vi "Subvi_Online_SVM_SWLDA_newMethod_in_분석기.vi"(0 "rate":dbl=500.0 caption="Rate" format="%0.2f", 1 "samples per channel":i32=25, 2 "in":T1, 4 "Brain_data_source":dbl[][](array[numeric]) caption="EEG_Raw_Data" format="%0.3f", 5 "Target_Flash_Order":i64[][](array[numeric]), 6 "Value":T1, 7 "svm_model_file":string, 8 "Matrix":T1, 10 "Target":path, 12 "Nontarget":path) -> (13 "EPR_발생_total":i16[](array[numeric]), 14 "output-0~8":i32, 15 "decision":dbl[](array[numeric]), 18 "SWLDA":dbl[](array[numeric]), 19 "ERP_Parameters":dbl[][](array[numeric]))   [LabVIEW 2014]
uses:
  <vilib>/Analysis/Matrix/Datatypes/RealMatrix.ctl
  <vilib>/Analysis/3filter.llb/Filter Passband Type.ctl
  <vilib>/Analysis/baseanly.llb/Mean (DBL).vi
  <vilib>/Analysis/3filter.llb/Butterworth Filter (DBL).vi
  <vilib>/Utility/file.llb/Read From Spreadsheet File (DBL).vi
  <vilib>/Analysis/Matrix/Numeric/Conversions/Array To Matrix - RA.vi
  <vilib>/Analysis/Matrix/Numeric/Multiply/Multiply - RM,RM.vi
  <vilib>/Analysis/Matrix/Numeric/Subtract/Subtract - RM,RM.vi
  <vilib>/Analysis/Matrix/Numeric/Conversions/Matrix To Array - RM.vi
  <vilib>/Analysis/NI_AALBase.lvlib
  <vilib>/Analysis/Matrix/NI_Matrix.lvlib
  <vilib>/Analysis/Matrix/Numeric/Conversions/Array To Matrix - RA2.vi
panel:
  out "Real":dbl
  out "deleted portion":dbl[][](array[numeric])
  out "2-D Array of Real 3":dbl[][](array[numeric])
  out "2-D Array of Real 2":dbl[][](array[numeric])
  out "2-D Array of Real":dbl[][](array[numeric])
  out "1-D Array of Real":dbl[](array[numeric])
  out "SWLDA_original":dbl[][](array[numeric])
  out "size(s)":i32[](array[numeric])
  in  "LDA":path=path "C:/Users/Administrator/Desktop/공공복지안전사업연구-노수진/파일럿20130902/LDA_Matrix_Value.xls"
  out "전치된 배열":dbl[][](array[numeric])
  out "#channel":i32
  out "#sti 6":i32
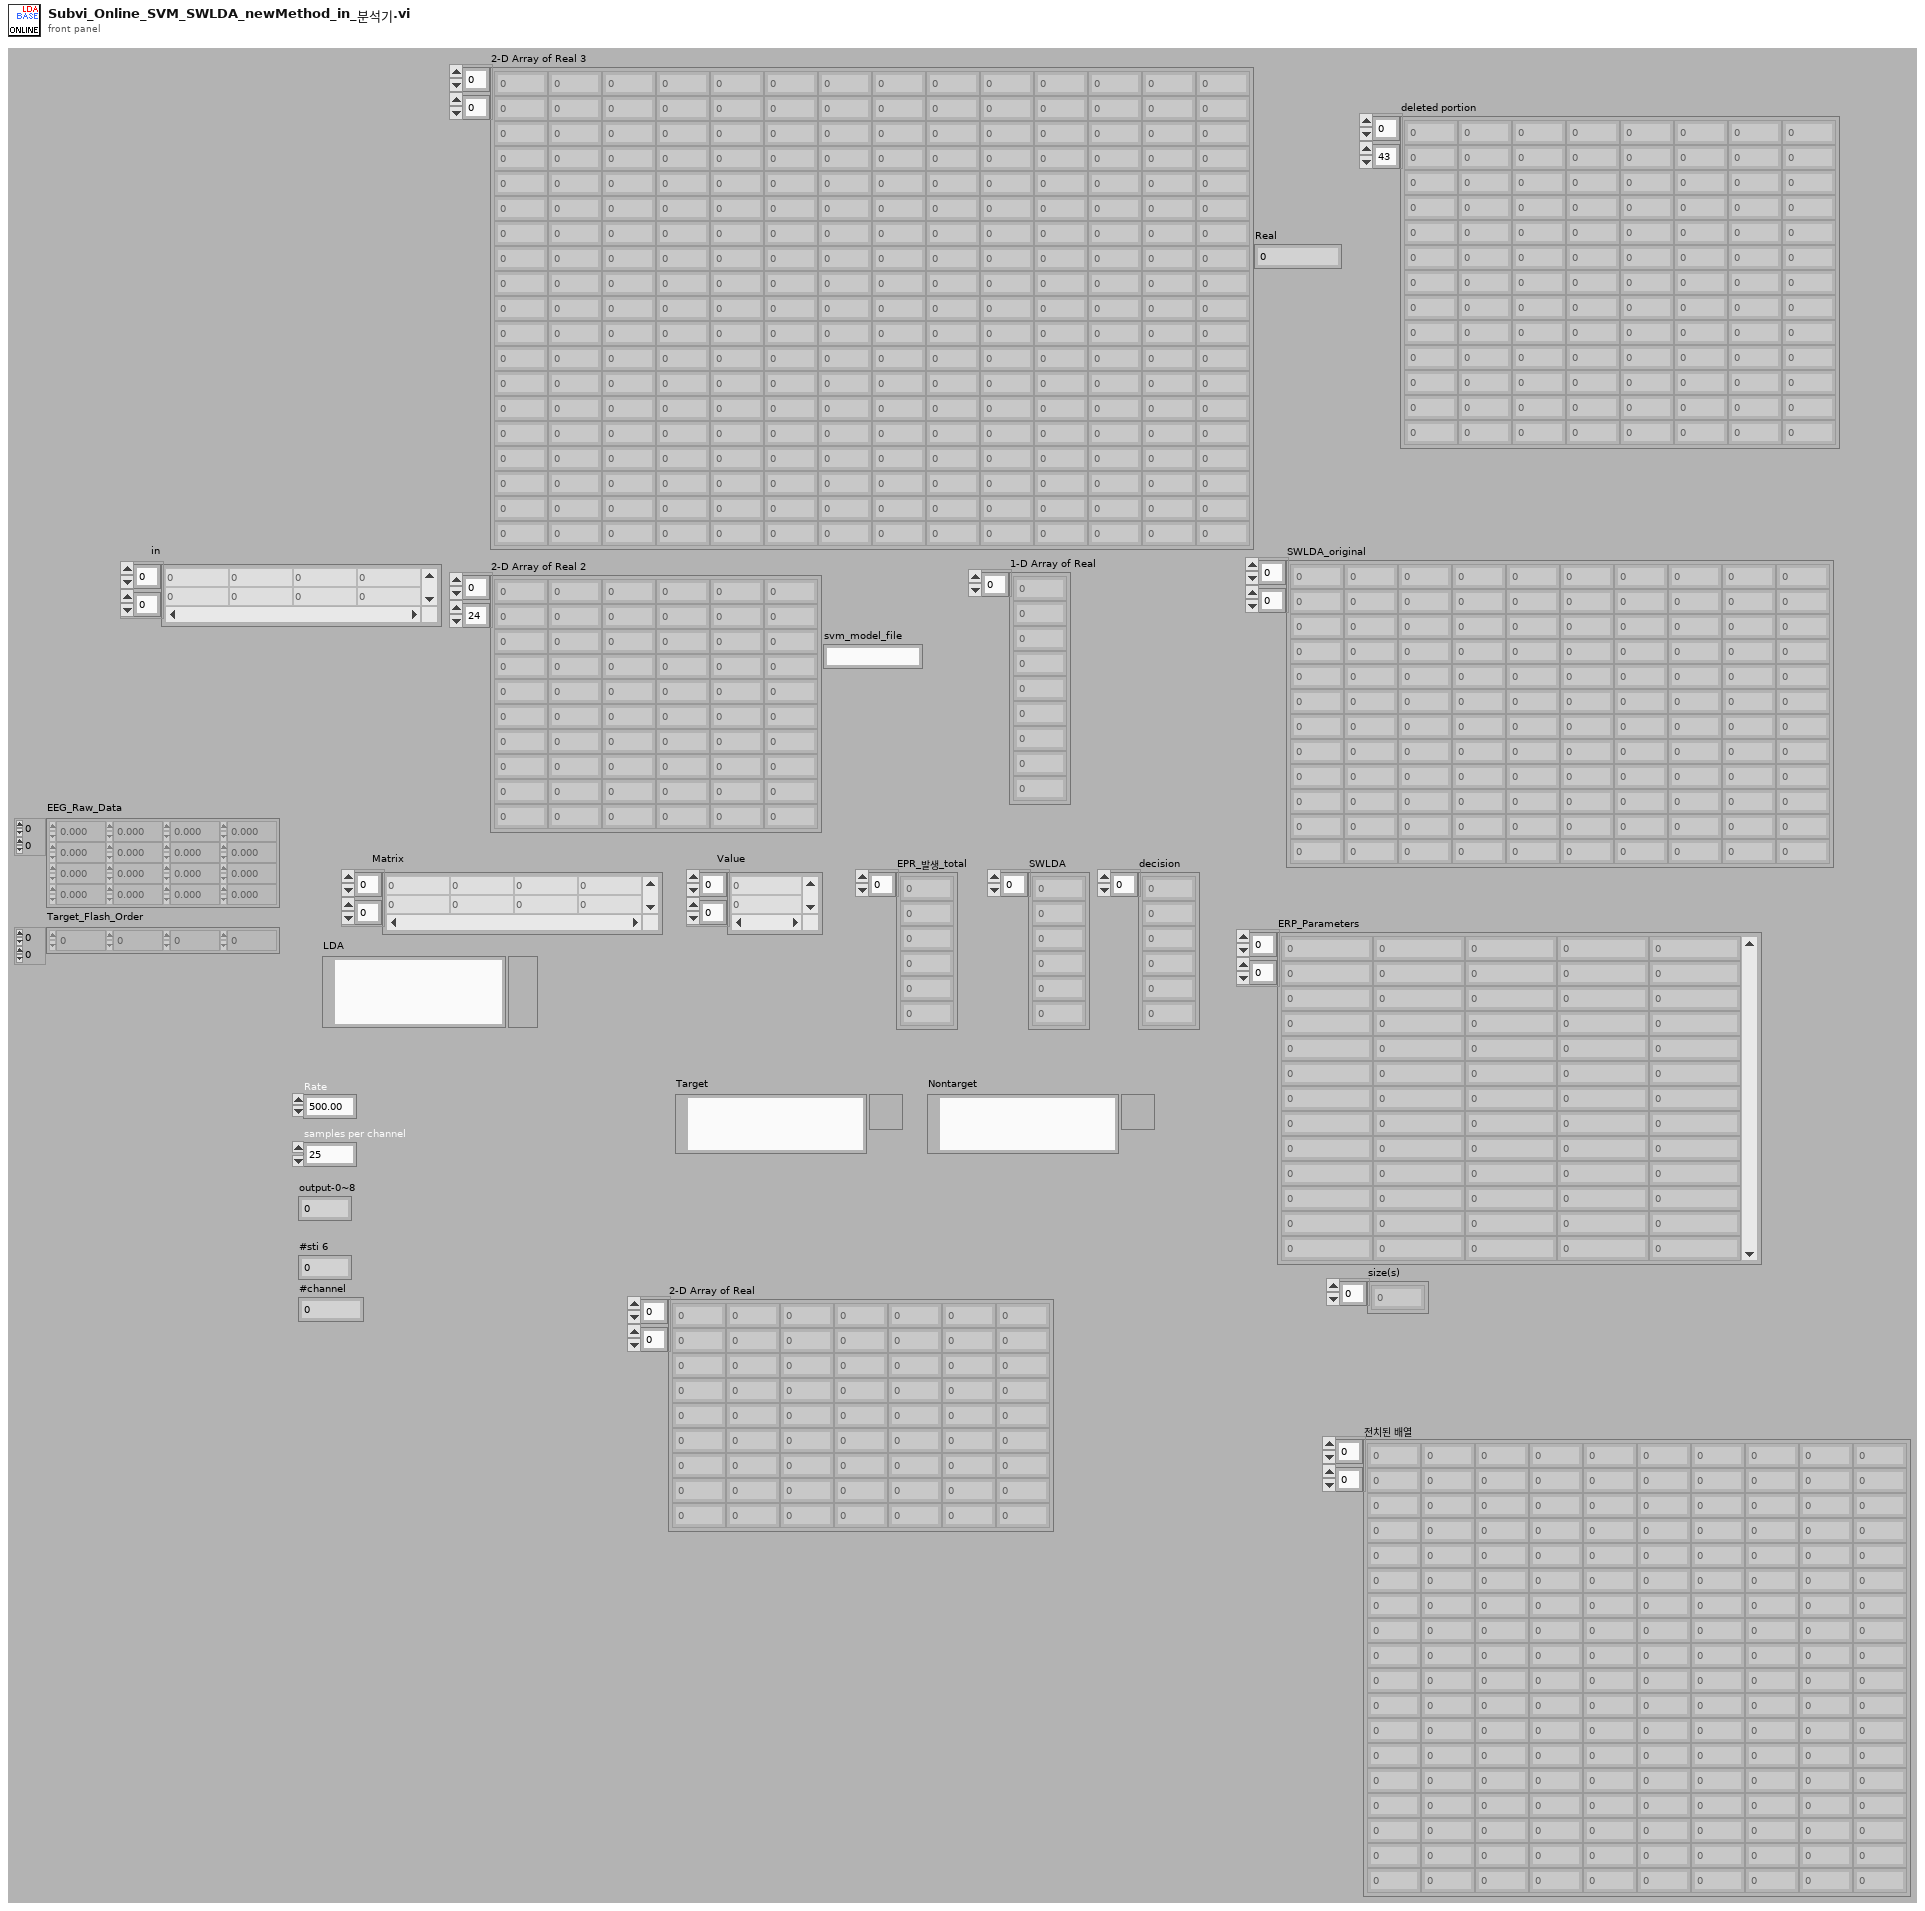
[diagram p1: front panel]
types:
  T1 = typedef "NI_Matrix.lvlib/RealMatrix.ctl" = dbl[][]
  T2 = typedef "NI_AALBase.lvlib/Filter Passband Type.ctl" = enum32{"Lowpass", "Highpass", "Bandpass", "Bandstop"}
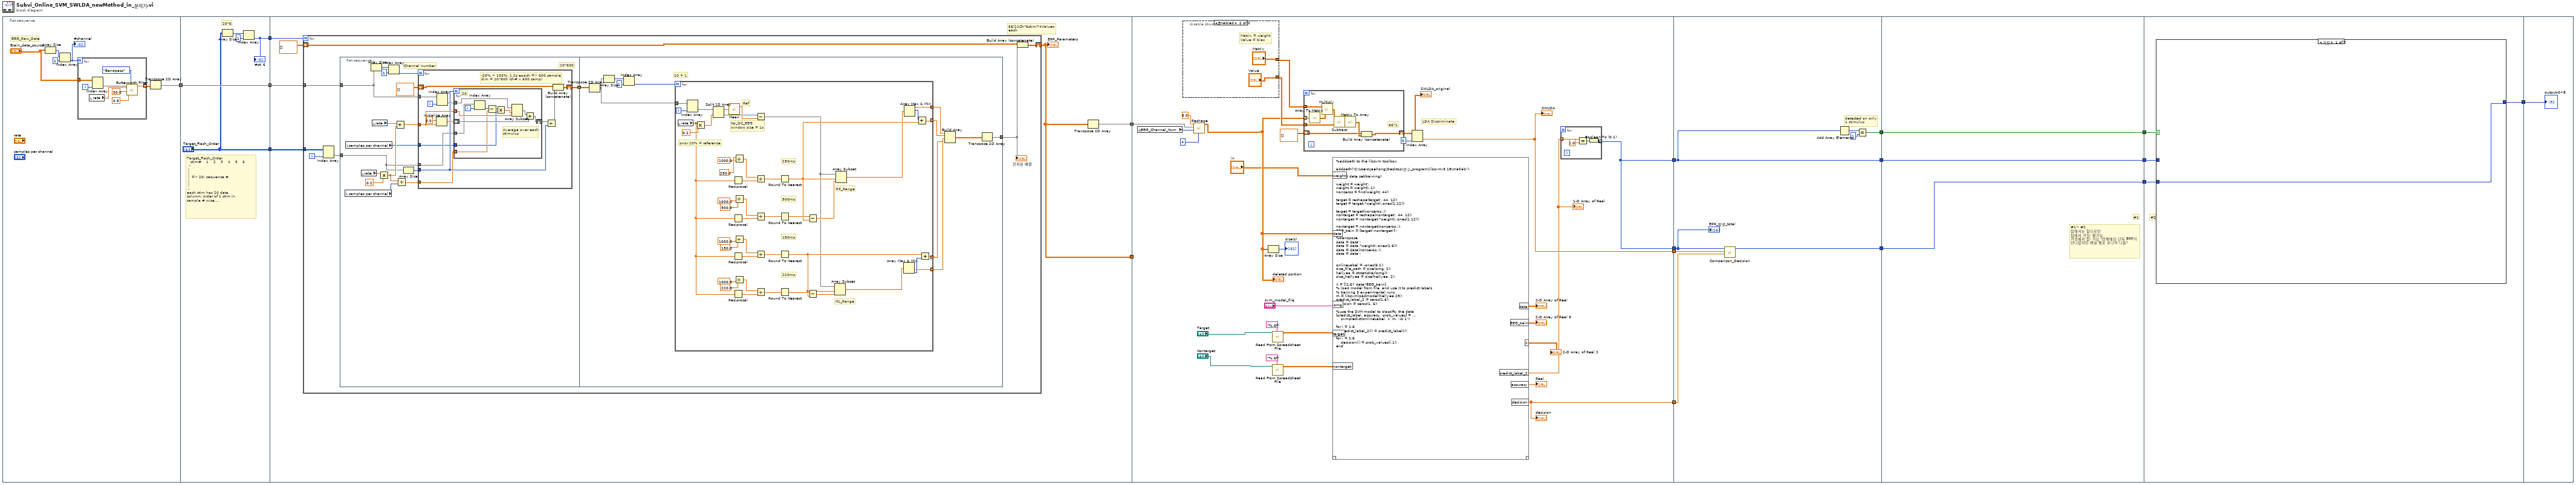
[diagram p0: block diagram]
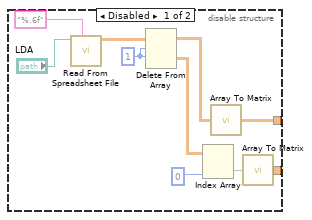
[diagram p2: hidden frame]
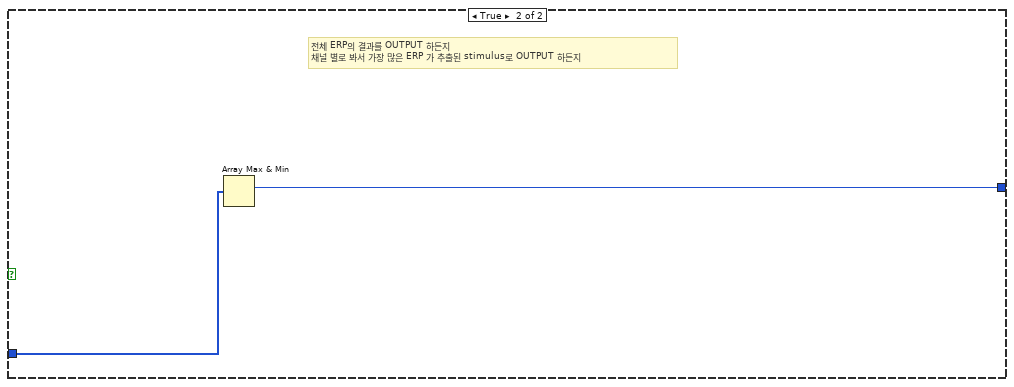
[diagram p3: hidden frame]
diagram:
  n1 = flat-sequence {
    tunnel: [w19] -> w17
    tunnel: [w36] -> w16
    tunnel: ["Target_Flash_Order"] -> w15
    tunnel: w17 -> [w36]
    tunnel: [w33] -> w14
    tunnel: w16 -> [w42]
    tunnel: w15 -> [w41]
    tunnel: w14 -> [w40]
    tunnel: [w37] -> w13
    tunnel: [w38] -> w12
    tunnel: w13 -> [w157]
    tunnel: w12 -> [_]
    tunnel: [w171] -> w11
    tunnel: [w171] -> w9
    tunnel: [w168] -> w7
    tunnel: [w152] -> w3
    tunnel: w11 -> [w204]
    tunnel: [w205] -> w10
    tunnel: w9 -> [w203]
    tunnel: w7 -> [w202]
    tunnel: [w204] -> w6
    tunnel: w3 -> [w201]
    tunnel: [w200] -> w2
    tunnel: w10 -> [w209]
    tunnel: w6 -> [w210]
    tunnel: [w210] -> w5
    tunnel: [w209] -> w4
    tunnel: w2 -> [w208]
    tunnel: [w208] -> w1
    tunnel: [w214] -> w8
    tunnel: w5 -> [w212]
    tunnel: w4 -> [w213]
    tunnel: w1 -> [w211]
    tunnel: w8 -> [w218]
    frame #0 {
      # "EEG_Raw_Data"
      n2 = Array Size(array="Brain_data_source") -> (size(s)=w20:i32[])
      n3 = Index Array(array=w20, index=1) -> (element=w22:i32)
      "#channel" <- w22
      n4 = for {
        N: w22 -> [_]
        tunnel: "Brain_data_source" -> [w31]
        tunnel: [w27] -> w23 mode=indexing
        i -> [w30]
        n5 = local read "rate"() -> (w24:dbl)
        n6 = Index Array(array=w31, index (col)=w30) -> (element=w29:dbl[])  [unwired: 1 in]
        n7 = call-poly <vilib>:"Butterworth Filter.vi"("filter type"=Filter_Passband_Type."Bandpass", "low cutoff freq: fl"=0.5, "high cutoff freq: fh"=30.0, "sampling freq: fs"=w24, "X"=w29) -> ("Filtered X"=w27:dbl[])  [unwired: 3 in, 1 out]
      }
      n8 = Transpose 2D Array(2D array=w23) -> (transposed array=w19:dbl[][])
    }
    frame #1 {
      # "Target_Flash_Order\n   stim#    1    2    3    4    5    6    \n  -\n |\n |\n |  => 20: sequence # \n |\n |\n -\neach stim has 20 data\ncolumn: order of 1 stim in \nsample # wise...."
      # "20*6"
      n9 = Array Size(array="Target_Flash_Order") -> (size(s)=w35:i32[])
      n10 = Index Array(array=w35, index=1 ("인덱스")) -> (element=w33:i32)
      "#sti 6" <- w33
    }
    frame #2 {
      # "66(11Ch*6stim)*4Values\neach"
      n11 = for {
        N: w40 -> [_]
        tunnel: w42 -> [w49]
        tunnel: w41 -> [w48]
        shift-right: [w45] -> w38
        shift-left: dbl[][] [] -> [w44]
        i -> [w47]
        n12 = Index Array(array=w48, index (col)=w47) -> (element=w46:i64[])  [unwired: 1 in]
        n13 = flat-sequence {
          tunnel: w49 -> [w53]
          tunnel: w46 -> [w52]
          tunnel: [w51] -> w50
          tunnel: w50 -> [w97]
          tunnel: [w93] -> w43
          frame #0 {
            # "10*600"
            # "Channel number"
            n14 = local read "samples per channel"() -> (w60:i32)
            n15 = local read "samples per channel"() -> (w59:i32)
            n16 = local read "rate"() -> (w62:dbl)
            n17 = Array Size(array=w53) -> (size(s)=w56:i32[])
            n18 = local read "rate"() -> (w64:dbl)
            n19 = Multiply(x=w62, y=0.2) -> (x*y=w66:dbl)
            n20 = Index Array(array=w56, index=1) -> (element=w58:i32)
            n21 = Add(x=w64, y=w66) -> (x+y=w65:dbl)
            n22 = Divide(x=w66, y=w60) -> (x/y=w63:dbl)
            n23 = Array Size(array=w52) -> (size(s)=w55:i32)
            n24 = for {
              N: w58 -> [_]
              tunnel: w59 -> [w67]
              tunnel: w65 -> [w78]
              shift-right: [w71] -> w51
              shift-left: dbl[][] [] -> [w73]
              tunnel: w55 -> [w72]
              tunnel: w53 -> [w70]
              tunnel: w52 -> [w69]
              tunnel: w63 -> [w68]
              i -> [w80]
              # "-20% ~ 100%: 1.2s epoch => 600 sample\ndim = 10*600 (ch# x 600 samp)"
              n25 = Initialize Array(0.0 ("element"), w78) -> (w77:dbl[])
              n26 = Index Array(array=w70, index (col)=w80) -> (element=w79:dbl[])  [unwired: 1 in]
              n27 = for {
                N: w72 -> [_]
                tunnel: w79 -> [w92]
                shift-right: [w89] -> w75
                shift-left: w77 -> [w90]
                tunnel: w78 -> [w88]
                tunnel: w69 -> [w86]
                tunnel: w68 -> [w84]
                tunnel: w67 -> [w82]
                i -> [w87]
                # "Average over each\nstimulus"
                # "20"
                n28 = Index Array(array=w86, index=w87) -> (element=w85:i64)
                n29 = Subtract(x=w85, y=w84) -> (x-y=w83:dbl)
                n30 = Multiply(x=w83, y=w82) -> (x*y=w81:dbl)
                n31 = Array Subset(array=w92, index=w81, length=w88) -> (w91:dbl[])
                n32 = Add(x=w91, y=w90) -> (x+y=w89:dbl[])
              }
              n33 = Divide(x=w75, y=w72) -> (x/y=w74:dbl[])
              n34 = Build Array (concatenate)(w73, w74) -> (w71:dbl[][])
            }
          }
          frame #1 {
            # "10 + 1"
            n35 = Transpose 2D Array(2D array=w97) -> (transposed array=w95:dbl[][])
            n36 = Array Size(array=w95) -> (size(s)=w98:i32[])
            n37 = Index Array(array=w98, index=1) -> (element=w94:i32)
            n38 = for {
              N: w94 -> [_]
              tunnel: w95 -> [w147]
              tunnel: [w142] -> w102 mode=indexing
              tunnel: [w140] -> w101 mode=indexing
              tunnel: [w111] -> w100 mode=indexing
              tunnel: [w137] -> w99 mode=indexing
              i -> [w136]
              # "P3_Range"
              # "N1_Range"
              # "220ms"
              # "150ms"
              # "500ms"
              # "250ms"
              # "No_DC_EEG\nwindow size = 1s"
              # "Ref"
              # "prior 20% = reference"
              n39 = local read "rate"() -> (w118:dbl)
              n40 = Index Array(array=w147, index (col)=w136) -> (element=w139:dbl[])  [unwired: 1 in]
              n41 = Multiply(x=w118, y=0.2) -> (x*y=w145:dbl)
              n42 = Split 1D Array(array=w139, index=w145) -> (first subarray=w144:dbl[], second subarray=w135:dbl[])
              n43 = call-poly <vilib>:"Mean.vi"("X"=w144) -> ("mean"=w143:dbl)  [unwired: 1 out]
              n44 = Reciprocal(x=w118) -> (1/x=w134:dbl)
              n45 = Reciprocal(x=w118) -> (1/x=w133:dbl)
              n46 = Reciprocal(x=w118) -> (1/x=w132:dbl)
              n47 = Reciprocal(x=w118) -> (1/x=w131:dbl)
              n48 = Divide(x=250.0, y=1000.0) -> (x/y=w130:dbl)
              n49 = Divide(x=500.0, y=1000.0) -> (x/y=w129:dbl)
              n50 = Divide(x=150.0, y=1000.0) -> (x/y=w128:dbl)
              n51 = Divide(x=220.0, y=1000.0) -> (x/y=w127:dbl)
              n52 = Subtract(x=w135, y=w143) -> (x-y=w104:dbl[])
              n53 = Divide(x=w130, y=w134) -> (x/y=w117:dbl)
              n54 = Divide(x=w129, y=w133) -> (x/y=w116:dbl)
              n55 = Divide(x=w128, y=w132) -> (x/y=w115:dbl)
              n56 = Divide(x=w127, y=w131) -> (x/y=w114:dbl)
              n57 = Round To Nearest(number=w117) -> (nearest integer value=w107:dbl)
              n58 = Round To Nearest(number=w116) -> (nearest integer value=w113:dbl)
              n59 = Round To Nearest(number=w115) -> (nearest integer value=w109:dbl)
              n60 = Round To Nearest(number=w114) -> (nearest integer value=w112:dbl)
              n61 = Subtract(x=w113, y=w107) -> (x-y=w108:dbl)
              n62 = Subtract(x=w112, y=w109) -> (x-y=w110:dbl)
              n63 = Array Subset(array=w104, index=w109, length=w110) -> (w105:dbl[])
              n64 = Array Subset(array=w104, index=w107, length=w108) -> (w106:dbl[])
              n65 = Array Max & Min(array=w105) -> (min value=w111:dbl, min index (indices)=w138:i32)  [unwired: 2 out]
              n66 = Array Max & Min(array=w106) -> (max value=w142:dbl, max index (indices)=w141:i32)  [unwired: 2 out]
              n67 = Add(x=w141, y=w107) -> (x+y=w140:dbl)
              n68 = Add(x=w109, y=w138) -> (x+y=w137:dbl)
            }
            n69 = Build Array(w102, w101, w100, w99) -> (w96:dbl[][])
            n70 = Transpose 2D Array(2D array=w96) -> (transposed array=w93:dbl[][])
          }
        }
        n71 = Build Array (concatenate)(w44, w43) -> (w45:dbl[][])
        "전치된 배열" <- w43
      }
      "ERP_Parameters" <- w38
      n72 = Transpose 2D Array(2D array=w38) -> (transposed array=w37:dbl[][])
    }
    frame #3 {
      # "LDA Discriminate"
      # "66*1"
      n73 = global read "Control_Panel_정리.vi" "EEG_Channel_Num"() -> (w156:i32)
      n74 = disable-structure shown="Enabled" {
        disable-tunnel: [w179 "Matrix"] -> w169
        disable-tunnel: [w178 "Value"] -> w170
        frame Disabled {
          w181 = 1 ("인덱스 (행)")
          n75 = call-poly <vilib>:"Read From Spreadsheet File.vi"("format (%.3f)"="%.6f", "file path (dialog if empty)"="LDA") -> ("all rows"=w175:dbl[][])  [unwired: 5 in, 4 out]
          n76 = Delete From Array(array=w175, length=w181, index (row)=w181) -> (deleted portion=w184:dbl[][], array with subset deleted=w183:dbl[][])  [unwired: 1 in]
          n77 = Index Array(array=w184, index (col)=0 ("인덱스")) -> (element=w182:dbl[])  [unwired: 1 in]
          n78 = call-poly <vilib>:"Array To Matrix.vi"("Real 2D Array"=w183) -> ("Real Matrix"=w179:T1)
          n79 = call-poly <vilib>:"Array To Matrix.vi"("Real 1D Array"=w182) -> ("Real Matrix (Column Vector)"=w178:T1)
        }
        frame Enabled {
          # "Matrix = weight\nValue = bias"
        }
      }
      n80 = call "Reshape.vi"("Numeric"=4, "EEG_Channel_Num"=w156, "all rows"=w157, "Numeric 2"=6.0) -> ("Array"=w153:dbl[][])  [unwired: 7 in]
      "deleted portion" <- w153
      n81 = Array Size(array=w153) -> (size(s)=→"size(s)":i32[])
      n82 = call-poly <vilib>:"Read From Spreadsheet File.vi"("format (%.3f)"="%.6f", "file path (dialog if empty)"="Target") -> ("all rows"=w165:dbl[][])  [unwired: 5 in, 4 out]
      n83 = call-poly <vilib>:"Read From Spreadsheet File.vi"("format (%.3f)"="%.6f", "file path (dialog if empty)"="Nontarget") -> ("all rows"=w164:dbl[][])  [unwired: 5 in, 4 out]
      n84 = for {
        tunnel: w169 -> [w191]
        tunnel: w170 -> [w197]
        shift-right: [w194] -> w172
        shift-left: dbl[][] [] -> [w193]
        tunnel: w153 -> [w192] mode=indexing
        n85 = call-poly <vilib>:"Array To Matrix.vi"("Real 1D Array"=w192) -> ("Real Matrix (Column Vector)"=w196:T1)
        n86 = call-poly <vilib>:"Multiply.vi"("Real Matrix B"=w196, "Real Matrix A"=w191) -> ("A * B"=w199:T1)
        n87 = call-poly <vilib>:"Subtract.vi"("Real Matrix B"=w197, "Real Matrix A"=w199) -> ("A - B"=w198:T1)
        n88 = call-poly <vilib>:"Matrix To Array.vi"("Real Matrix"=w198) -> ("Real 2D Array"=w195:dbl[][])
        n89 = Build Array (concatenate)(w193, w195) -> (w194:dbl[][])
      }
      "SWLDA_original" <- w172
      n90 = script code="%addpath to the libsvm toolbox\n\naddpath('C:\\Users\\Jaehong\\Desktop\\연구_program\\libsvm-3.18\\matlab');\n\n%read data set(training)\n\nweight = weight';\nweight = weight(:,1);\nnonzeros = find(weight, 44);\n\ntarget = reshape(target', 44, 12);\ntarget = target.*weight(:,ones(1,12));\n\ntarget = target(nonzeros,:);\nnontarget = reshape(nontarget', 44, 12);\nnontarget = nontarget.*weight(:,ones(1,12));\n\nnontarget = nontarget(nonzeros,:);\nEEG_train = [target';nontarget']';\n\n%transpose\ndata = data';\ndata = data.*weight(:,ones(1,6));\ndata = data(nonzeros,:);\ndata = data';\n\n\nonlineLabel = -ones(6,1);\nsize_file_path = size(omg, 2);\nhellyea = strcat(char(omg));\nsize_hellyea = size(hellyea, 2);\n\nX = [(1:6)' data*EEG_train];\n% load model from file, and use it to predict labels\n% training 3 experimental runs\nm = libsvmloadmodel(hellyea,25);\npredict_label_2 = zeros(1,6);\ndecision = zeros(1, 6);\n\n%use the SVM model to classifty the data\n[predict_label, accuracy, prob_values] = ...\n    svmpredict(onlineLabel, X, m, '-b 1');\n\nfor i = 1:6\n    predict_label_2(i) = predict_label(i);\nend\nfor i = 1:6\n    decision(i) = prob_values(i,1);\nend"("weight"="in", "target"=w165, "nontarget"=w164, "data"=w153, "omg"="svm_model_file") -> ("predict_label_2"=w163:dbl[], "data"=→"2-D Array of Real":dbl[][], "EEG_train"=→"2-D Array of Real 3":dbl[][], "X"=→"2-D Array of Real 2":dbl[][], "accuracy"=→"Real":dbl, "decision"=w152:dbl[])  [unwired: 1 in, 1 out]
      "1-D Array of Real" <- w163
      "decision" <- w152
      n91 = Index Array(array=w172, index (col)=0 ("비활성화된 인덱스 (열)")) -> (element=w168:dbl[])  [unwired: 1 in]
      "SWLDA" <- w168
      n92 = for {
        tunnel: w163 -> [w190] mode=indexing
        tunnel: [w189] -> w171 mode=indexing
        n93 = Equal?(x=w190, y=1.0) -> (x = y?=w187:bool)
        n94 = Boolean To (0,1)(Boolean=w187) -> (0, 1=w189:i16)
      }
    }
    frame #4 {
      # "detected on only\n1 stimulus"
      n95 = call "Comparison_Decision.vi"("decision"=w201, "SWLDA"=w202, "EPR_발생_total"=w203) -> ("selected"=w200:i32)  [unwired: 8 in]
      n96 = Add Array Elements(numeric array=w204) -> (sum=w207:i16)
      n97 = Equal?(x=w207, y=i16 1) -> (x = y?=w205:bool)
      "EPR_발생_total" <- w203
    }
    frame #5 {
      # "#1> #2\n참에서는 참으로만\n참에서 거짓: 불가능\n거짓에서 참: 가능 (전체에선 단독 ERP가 안나왔지만 채널 별로 보니까 나옴)"
      # "#1"
    }
    frame #6 {
      # "#2"
      n98 = case shown="거짓" w213 {
        tunnel: [w215 w217] -> w214
        tunnel: w212 -> [_ w216]
        tunnel: w211 -> [w215 _]
        frame False {
        }
        frame True {
          # "전체 ERP의 결과를 OUTPUT 하든지\n채널 별로 봐서 가장 많은 ERP 가 추출된 stimulus로 OUTPUT 하든지"
          n99 = Array Max & Min(array=w216) -> (max index (indices)=w217:i32)  [unwired: 3 out]
        }
      }
    }
    frame #7 {
      "output-0~8" <- w218
    }
  }
